vi "SetPaneSize.vi"(8 "error in (no error)":errorcluster, 9 "Pane Size":i32, 10 "Pane Position":T1 items=["Top", "Left", "Center", "Right", "Bottom"], 11 "PentaPanesGUI in":refnum<class "PentaPanes.lvclass">) -> (0 "error out":errorcluster, 3 "PentaPanesGUI out":refnum<class "PentaPanes.lvclass">)   [LabVIEW 2022 SP3, in "PentaPanesLibrary.lvlib" / "PentaPanes.lvclass"]
doc: "SetPaneSize\nThis vi changes the size of a specified pane identified by its position. \n\nPane Position - Selects the pane to be resized by its position (top, left, right and bottom) \nPane Size - The size that the pane is set to. (in pixels)"
uses:
  PentaPanes.lvclass
  PanePosition.ctl
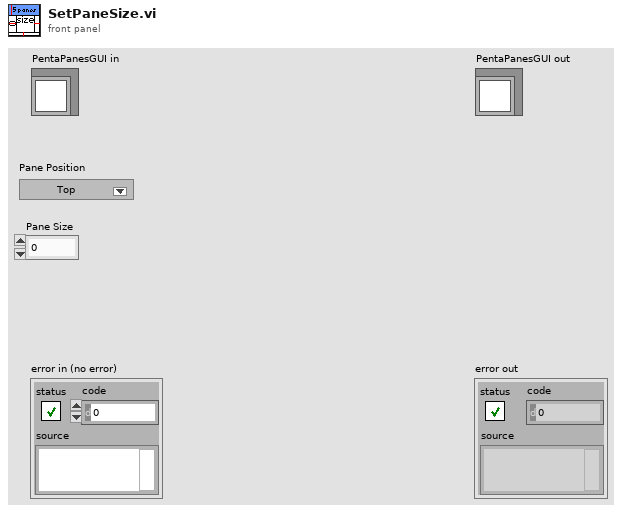
[diagram p1: front panel]
types:
  T1 = typedef "PentaPanesLibrary.lvlib/PentaPanes.lvclass/PanePosition.ctl" = u16
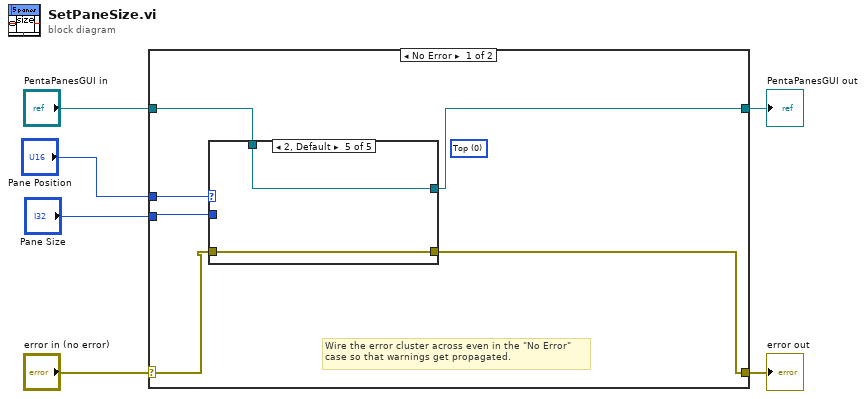
[diagram p0: block diagram]
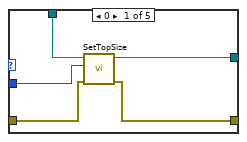
[diagram p2: hidden frame]
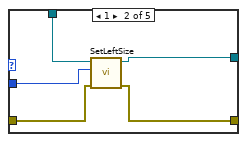
[diagram p3: hidden frame]
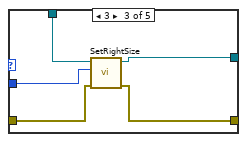
[diagram p4: hidden frame]
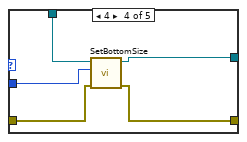
[diagram p5: hidden frame]
diagram:
  n1 = case shown="No Error" "error in (no error)" {
    selector: "error in (no error)" -> [w9 w36]
    tunnel: [w8 w36] -> w5
    tunnel: [w7 w35] -> w3
    tunnel: "PentaPanesGUI in" -> [w12 w35]
    tunnel: "Pane Size" -> [w11 _]
    tunnel: "Pane Position" -> [w10 _]
    frame No Error {
      (unwired) T1 0 items=["Top", "Left", "Center", "Right", "Bottom"] ("Position")
      # "Wire the error cluster across even in the \"No Error\"\ncase so that warnings get propagated."
      n2 = case shown="2, Default" w10 {
        tunnel: w12 -> [w17 w22 w27 w32 w34]
        tunnel: w11 -> [w16 w18 w23 w28 _]
        tunnel: w9 -> [w15 w19 w24 w29 w33]
        tunnel: [w14 w20 w25 w30 w33] -> w8
        tunnel: [w13 w21 w26 w31 w34] -> w7
        frame 0 {
          n3 = call-dynamic "SetTopSize.vi"("error in (no error)"=w15, "Top Pane Size"=w16, "PentaPanesGUI in"=w17) -> ("error out"=w14:errorcluster, "PentaPanesGUI out"=w13:refnum<class "PentaPanes.lvclass">)  [unwired: 7 in]
        }
        frame 1 {
          n4 = call-dynamic "SetLeftSize.vi"("error in (no error)"=w19, "Left Pane Size"=w18, "PentaPanesGUI in"=w22) -> ("error out"=w20:errorcluster, "PentaPanesGUI out"=w21:refnum<class "PentaPanes.lvclass">)  [unwired: 7 in]
        }
        frame 3 {
          n5 = call-dynamic "SetRightSize.vi"("error in (no error)"=w24, "Right Pane Size"=w23, "PentaPanesGUI in"=w27) -> ("error out"=w25:errorcluster, "PentaPanesGUI out"=w26:refnum<class "PentaPanes.lvclass">)  [unwired: 7 in]
        }
        frame 4 {
          n6 = call-dynamic "SetBottomSize.vi"("error in (no error)"=w29, "Bottom Pane Size"=w28, "PentaPanesGUI in"=w32) -> ("error out"=w30:errorcluster, "PentaPanesGUI out"=w31:refnum<class "PentaPanes.lvclass">)  [unwired: 7 in]
        }
        frame 2, Default {
        }
      }
    }
    frame Error {
    }
  }
  "error out" <- w5
  "PentaPanesGUI out" <- w3
